vi "check_is_moving.vi"(8 "error in (no error)":errorcluster, 11 "dummyStageRapid in":refnum<class "dummyStageRapid.lvclass">) -> (0 "error out":errorcluster, 2 "number":dbl, 3 "dummyStageRapid out":refnum<class "dummyStageRapid.lvclass">)   [LabVIEW 2019, in "dummyStageRapid.lvlib" / "dummyStageRapid.lvclass"]
uses:
  dummyStageRapid.lvclass
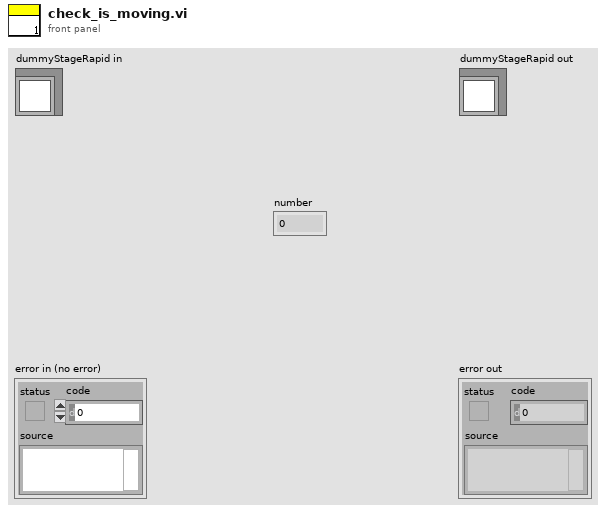
[diagram p1: front panel]
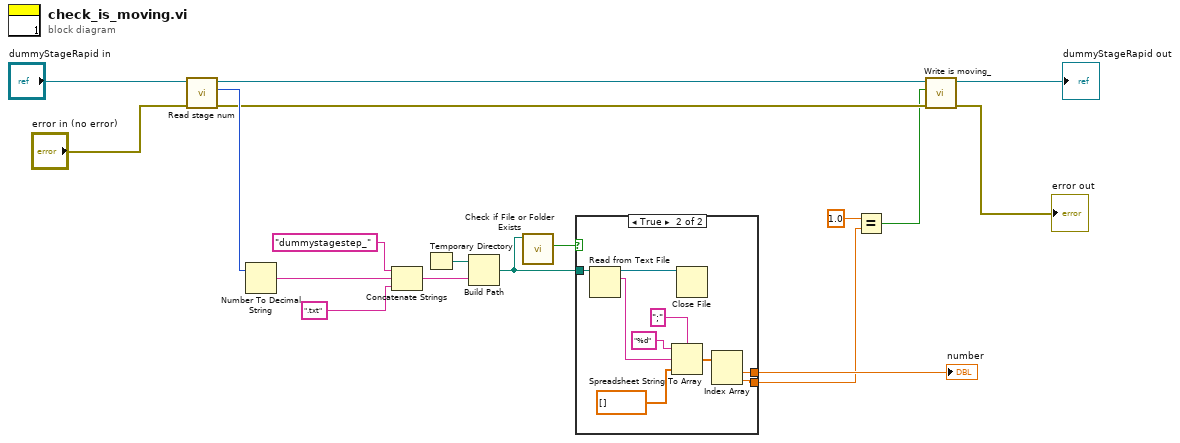
[diagram p0: block diagram]
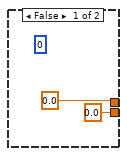
[diagram p2: hidden frame]
diagram:
  n1 = call-dynamic "Read stage num.vi"("error in (no error)"="error in (no error)", "_stage in"="dummyStageRapid in") -> ("error out"=w5:errorcluster, "stage num"=w10:u8, "_stage out"=w6:refnum<class "dummyStageRapid.lvclass">)  [unwired: 7 in]
  n2 = Number To Decimal String(number=w10) -> (decimal integer string=w17:string)  [unwired: 1 in]
  n3 = Concatenate Strings("dummystagestep_", w17, ".txt") -> (w15:string)
  n4 = Temporary Directory() -> (w14:path)
  n5 = Build Path(base path=w14, name or relative path=w15) -> (appended path=w13:path)
  n6 = call <vilib>:"Check if File or Folder Exists.vi"("path"=w13) -> ("file or folder exists?"=w12:bool)  [unwired: 8 in, 2 out]
  n7 = case shown="True" w12 {
    tunnel: w13 -> [_ w28]
    tunnel: [0.0 w22] -> w3
    tunnel: [0.0 w21] -> w2
    frame False {
      (unwired) 0
    }
    frame True {
      n8 = Read from Text File(file (use dialog)=w28) -> (refnum out=w29:refnum<file>, text=w26:string)  [unwired: 3 in, 2 out]
      n9 = Spreadsheet String To Array(delimiter (Tab)=";", format string="%d", spreadsheet string=w26, array type (2D Dbl)=dbl[] []) -> (array=w25:dbl[])
      n10 = Close File(refnum=w29) -> ()  [unwired: 1 in, 2 out]
      n11 = Index Array(array=w25) -> (element #1=w22:dbl, element #2=w21:dbl)  [unwired: 2 in]
    }
  }
  "number" <- w3
  n12 = Equal?(x=1.0, y=w2) -> (x = y?=w1:bool)
  n13 = call-dynamic "Write is moving_.vi"("error in (no error)"=w5, "is moving?"=w1, "_stage in"=w6) -> ("error out"=→"error out":errorcluster, "_stage out"=→"dummyStageRapid out":refnum<class "dummyStageRapid.lvclass">)  [unwired: 7 in]
